vi "SP Convert 2.2 to 3.0 - 3.1.vi"(1 "S Parameter 2.2 Test Parameters":T2={"Tag"="", "Stimulus"={"Use Instrument Settings"=FALSE, "Sweep Type"=enum."Linear", "Sweep"=[{"Fstart, MHz"=500.0, "Fstop, MHz"=1500.0, "Points"=201}], "Blank Frequencies"=FALSE, "Power, dBm"=999.0, "IFBW, Hz"=-1.0, "Sweep Time, s"=-1.0}, "Measurements"=[{"Parameter"=enum."S11", "Channel"=1, "Limits"=[]}], "Reports"={"Reports to Generate"=[], "Print Reports"=FALSE}, "Quick Mode"=FALSE, "Display"={"Retain Settings"=FALSE, "Lock Control"=FALSE, "Plot Orientation"=enum."Single", "CH Controls"=[{"Trace Orientation"=enum."Overlay", "Frequency"={"Start"=500.0, "Stop"=1500.0, "Units"="MHz"}, "CH1Control"={"ChOn"=TRUE, "Measure"=0, "Format"=0, "Autoscale"=TRUE, "Reference"=0.0, "\nRefUnit"="dB/Div", "Position"=5.0, "Scale"=10.0, "ScaleUnit"="dB/Div", "LimitOn"=TRUE, "LimitFill"=FALSE, "Display Data"=0}, "CH2Control"={"ChOn"=TRUE, "Measure"=0, "Format"=0, "Autoscale"=TRUE, "Reference"=0.0, "\nRefUnit"="dB/Div", "Position"=5.0, "Scale"=10.0, "ScaleUnit"="dB/Div", "LimitOn"=TRUE, "LimitFill"=FALSE, "Display Data"=0}}, {"Trace Orientation"=enum."Overlay", "Frequency"={"Start"=500.0, "Stop"=1500.0, "Units"="MHz"}, "CH1Control"={"ChOn"=TRUE, "Measure"=0, "Format"=0, "Autoscale"=TRUE, "Reference"=0.0, "\nRefUnit"="dB/Div", "Position"=5.0, "Scale"=10.0, "ScaleUnit"="dB/Div", "LimitOn"=TRUE, "LimitFill"=FALSE, "Display Data"=0}, "CH2Control"={"ChOn"=TRUE, "Measure"=0, "Format"=0, "Autoscale"=TRUE, "Reference"=0.0, "\nRefUnit"="dB/Div", "Position"=5.0, "Scale"=10.0, "ScaleUnit"="dB/Div", "LimitOn"=TRUE, "LimitFill"=FALSE, "Display Data"=0}}, {"Trace Orientation"=enum."Overlay", "Frequency"={"Start"=500.0, "Stop"=1500.0, "Units"="MHz"}, "CH1Control"={"ChOn"=TRUE, "Measure"=0, "Format"=0, "Autoscale"=TRUE, "Reference"=0.0, "\nRefUnit"="dB/Div", "Position"=5.0, "Scale"=10.0, "ScaleUnit"="dB/Div", "LimitOn"=TRUE, "LimitFill"=FALSE, "Display Data"=0}, "CH2Control"={"ChOn"=TRUE, "Measure"=0, "Format"=0, "Autoscale"=TRUE, "Reference"=0.0, "\nRefUnit"="dB/Div", "Position"=5.0, "Scale"=10.0, "ScaleUnit"="dB/Div", "LimitOn"=TRUE, "LimitFill"=FALSE, "Display Data"=0}}, {"Trace Orientation"=enum."Overlay", "Frequency"={"Start"=500.0, "Stop"=1500.0, "Units"="MHz"}, "CH1Control"={"ChOn"=TRUE, "Measure"=0, "Format"=0, "Autoscale"=TRUE, "Reference"=0.0, "\nRefUnit"="dB/Div", "Position"=5.0, "Scale"=10.0, "ScaleUnit"="dB/Div", "LimitOn"=TRUE, "LimitFill"=FALSE, "Display Data"=0}, "CH2Control"={"ChOn"=TRUE, "Measure"=0, "Format"=0, "Autoscale"=TRUE, "Reference"=0.0, "\nRefUnit"="dB/Div", "Position"=5.0, "Scale"=10.0, "ScaleUnit"="dB/Div", "LimitOn"=TRUE, "LimitFill"=FALSE, "Display Data"=0}}], "Formatted Data"=FALSE}, "Calibrations"=[enum."Not Calibrated", enum."Not Calibrated", enum."Not Calibrated", enum."Not Calibrated"]} {"Display"."CH Controls"."Frequency"."Stop" format="%.3g"; "Display"."CH Controls"."Frequency"."Start" format="%.3g"; "Display"."CH Controls"."CH2Control"."Measure" items=["S11", "S21", "S12", "S22"]; "Display"."CH Controls"."CH2Control"."Reference" format="%#.2g"; "Display"."CH Controls"."CH2Control"."Display Data" items=["Data", "Memory", "Data/Memory"]; "Display"."CH Controls"."CH2Control"."Format" items=["Log Mag", "Phase", "Delay", "Smith", "Polar", "Lin Mag", "SWR", "Loss", "Real", "Imaginary"]; "Display"."CH Controls"."CH2Control"."Scale" min=0.001 step=1.0 format="%#.2g"; "Display"."CH Controls"."CH2Control"."Position" min=0.0 max=10.0; "Display"."CH Controls"."CH1Control"."Measure" items=["S11", "S21", "S12", "S22"]; "Display"."CH Controls"."CH1Control"."Reference" format="%#.2g"; "Display"."CH Controls"."CH1Control"."Display Data" items=["Data", "Memory", "Data/Memory"]; "Display"."CH Controls"."CH1Control"."Format" items=["Log Mag", "Phase", "Delay", "Smith", "Polar", "Lin Mag", "SWR", "Loss", "Real", "Imaginary"]; "Display"."CH Controls"."CH1Control"."Scale" min=0.001 step=1.0 format="%#.2g"; "Display"."CH Controls"."CH1Control"."Position" min=0.0 max=10.0; "Stimulus"."Sweep Time, s" format="%.3g"; "Measurements"."Channel" min=1 max=99 step=1}) -> (0 "S Parameter 3.0 - 3.1 Test Parameters":T1={"Tag"="", "Stimulus"={"Use Instrument Settings"=FALSE, "Sweep Type"=enum."Linear", "Sweep"=[{"Fstart, MHz"=500.0, "Fstop, MHz"=1500.0, "Points"=201}], "Blank Frequencies"=FALSE, "Power, dBm"=999.0, "IFBW, Hz"=-1.0, "Sweep Time, s"=-1.0}, "Measurements"=[], "Reports"={"Reports to Generate"=[], "Print Reports"=FALSE}, "Quick Mode"=FALSE, "Display"={"Retain Settings"=TRUE, "Lock Control"=FALSE, "Plot Orientation"=enum."Single", "CH Controls"=[{"Trace Orientation"=enum."Overlay", "Frequency"={"Start"=500.0, "Stop"=1500.0, "Units"="MHz"}, "CH1Control"={"ChOn"=TRUE, "Measure"=0, "Format"=6, "Autoscale"=FALSE, "Reference"=0.0, "\nRefUnit"="dB/Div", "Position"=5.0, "Scale"=1.0, "ScaleUnit"="dB/Div", "LimitOn"=TRUE, "LimitFill"=FALSE, "Display Data"=0, "Show Markers"=FALSE}, "CH2Control"={"ChOn"=TRUE, "Measure"=0, "Format"=6, "Autoscale"=FALSE, "Reference"=0.0, "\nRefUnit"="dB/Div", "Position"=5.0, "Scale"=1.0, "ScaleUnit"="dB/Div", "LimitOn"=TRUE, "LimitFill"=FALSE, "Display Data"=0, "Show Markers"=FALSE}, "Markers"=[]}, {"Trace Orientation"=enum."Overlay", "Frequency"={"Start"=500.0, "Stop"=1500.0, "Units"="MHz"}, "CH1Control"={"ChOn"=TRUE, "Measure"=0, "Format"=6, "Autoscale"=TRUE, "Reference"=0.0, "\nRefUnit"="dB/Div", "Position"=5.0, "Scale"=1.0, "ScaleUnit"="dB/Div", "LimitOn"=TRUE, "LimitFill"=FALSE, "Display Data"=0, "Show Markers"=FALSE}, "CH2Control"={"ChOn"=TRUE, "Measure"=1, "Format"=0, "Autoscale"=TRUE, "Reference"=0.0, "\nRefUnit"="dB/Div", "Position"=5.0, "Scale"=1.0, "ScaleUnit"="dB/Div", "LimitOn"=TRUE, "LimitFill"=FALSE, "Display Data"=0, "Show Markers"=FALSE}, "Markers"=[]}, {"Trace Orientation"=enum."Overlay", "Frequency"={"Start"=500.0, "Stop"=1500.0, "Units"="MHz"}, "CH1Control"={"ChOn"=TRUE, "Measure"=0, "Format"=6, "Autoscale"=TRUE, "Reference"=0.0, "\nRefUnit"="dB/Div", "Position"=5.0, "Scale"=1.0, "ScaleUnit"="dB/Div", "LimitOn"=TRUE, "LimitFill"=FALSE, "Display Data"=0, "Show Markers"=FALSE}, "CH2Control"={"ChOn"=TRUE, "Measure"=1, "Format"=0, "Autoscale"=TRUE, "Reference"=0.0, "\nRefUnit"="dB/Div", "Position"=5.0, "Scale"=1.0, "ScaleUnit"="dB/Div", "LimitOn"=TRUE, "LimitFill"=FALSE, "Display Data"=0, "Show Markers"=FALSE}, "Markers"=[]}, {"Trace Orientation"=enum."Overlay", "Frequency"={"Start"=500.0, "Stop"=1500.0, "Units"="MHz"}, "CH1Control"={"ChOn"=TRUE, "Measure"=0, "Format"=6, "Autoscale"=TRUE, "Reference"=0.0, "\nRefUnit"="dB/Div", "Position"=5.0, "Scale"=1.0, "ScaleUnit"="dB/Div", "LimitOn"=TRUE, "LimitFill"=FALSE, "Display Data"=0, "Show Markers"=FALSE}, "CH2Control"={"ChOn"=TRUE, "Measure"=1, "Format"=0, "Autoscale"=TRUE, "Reference"=0.0, "\nRefUnit"="dB/Div", "Position"=5.0, "Scale"=1.0, "ScaleUnit"="dB/Div", "LimitOn"=TRUE, "LimitFill"=FALSE, "Display Data"=0, "Show Markers"=FALSE}, "Markers"=[]}], "Formatted Data"=FALSE}, "Calibrations"=[enum."Not Calibrated", enum."Not Calibrated", enum."Not Calibrated", enum."Not Calibrated"]} {"Stimulus"."Sweep Time, s" format="%.3g"; "Display"."CH Controls"."Frequency"."Stop" format="%.3g"; "Display"."CH Controls"."Frequency"."Start" format="%.3g"; "Display"."CH Controls"."CH2Control"."Measure" items=["S11", "S21", "S12", "S22"]; "Display"."CH Controls"."CH2Control"."Reference" format="%#.2g"; "Display"."CH Controls"."CH2Control"."Display Data" items=["Data", "Memory", "Data/Memory"]; "Display"."CH Controls"."CH2Control"."Format" items=["Log Mag", "Phase", "Delay", "Smith", "Polar", "Lin Mag", "SWR", "Loss", "Real", "Imaginary"]; "Display"."CH Controls"."CH2Control"."Scale" min=0.001 step=1.0 format="%#.2g"; "Display"."CH Controls"."CH2Control"."Position" min=0.0 max=10.0; "Display"."CH Controls"."CH1Control"."Measure" items=["S11", "S21", "S12", "S22"]; "Display"."CH Controls"."CH1Control"."Reference" format="%#.2g"; "Display"."CH Controls"."CH1Control"."Display Data" items=["Data", "Memory", "Data/Memory"]; "Display"."CH Controls"."CH1Control"."Format" items=["Log Mag", "Phase", "Delay", "Smith", "Polar", "Lin Mag", "SWR", "Loss", "Real", "Imaginary"]; "Display"."CH Controls"."CH1Control"."Scale" min=0.001 step=1.0 format="%#.2g"; "Display"."CH Controls"."CH1Control"."Position" min=0.0 max=10.0; "Measurements"."Channel" min=1 max=99 step=1; "Measurements"."Limits"."Run" min=1 step=1})   [LabVIEW 2011]
uses:
  TypeDefs/SP Test Parameters v2.2.ctl
  TypeDefs/SP Test Parameters v3.0-3.1.ctl
panel:
  # "Div"
  # "Div"
  # "="
  # "Div"
  # "Div"
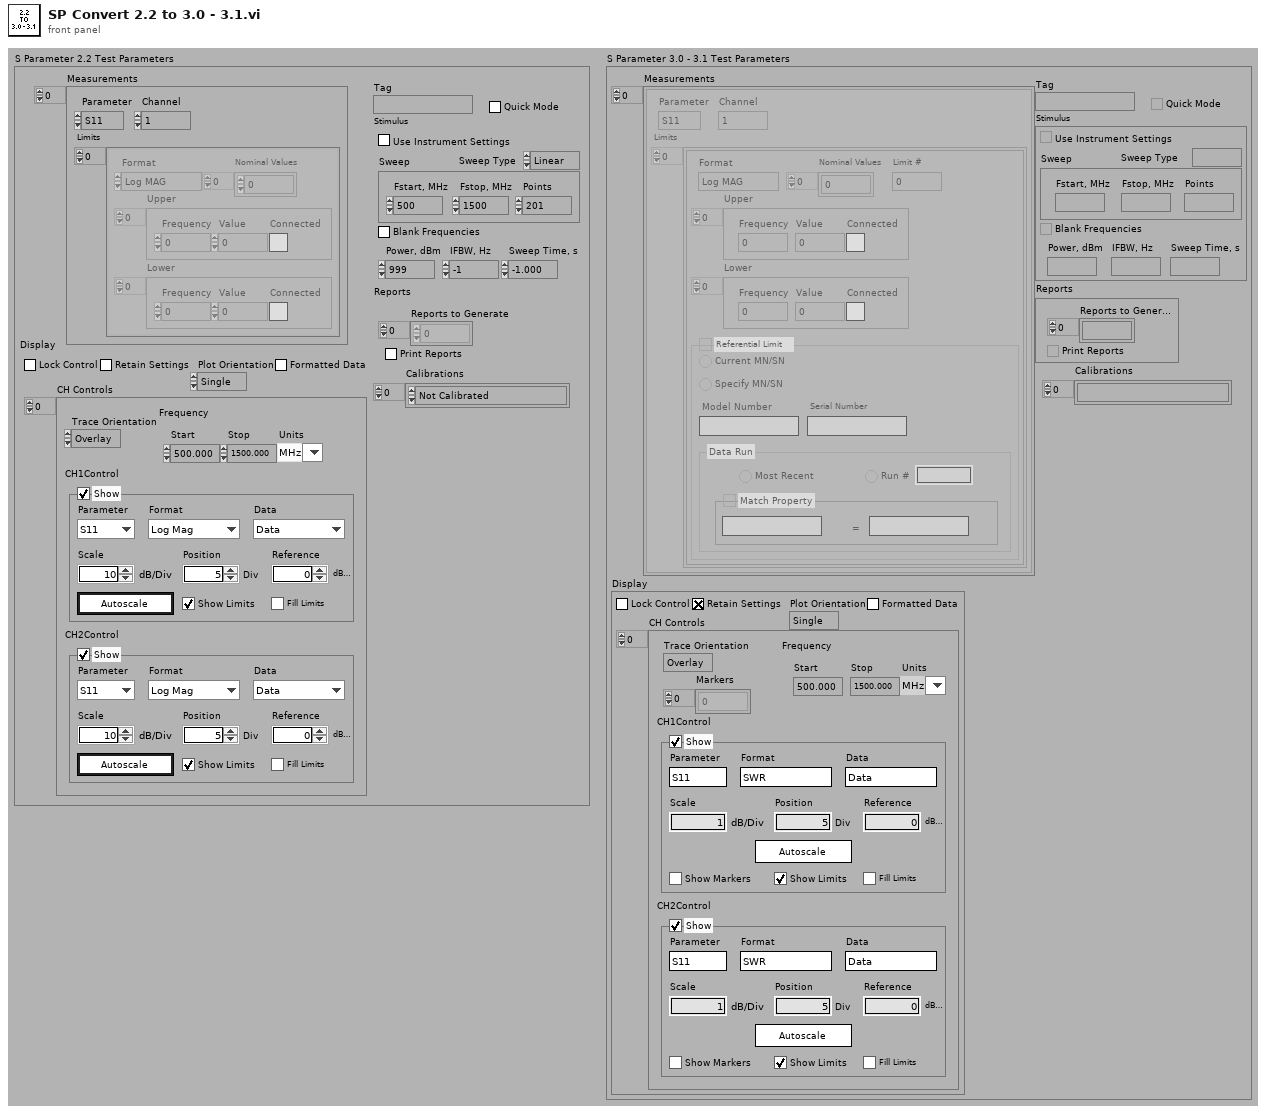
[diagram p1: front panel]
types:
  T1 = typedef "SP Test Parameters v3.0-3.1.ctl" = cluster{"Tag":string, "Stimulus":cluster{"Use Instrument Settings":bool, "Sweep Type":enum32{"Linear", "Log", "List", "Power", "CW"}, "Sweep":cluster{"Fstart, MHz":dbl, "Fstop, MHz":dbl, "Points":i32}[], "Blank Frequencies":bool, "Power, dBm":dbl, "IFBW, Hz":dbl, "Sweep Time, s":dbl}, "Measurements":cluster{"Parameter":enum32{"S11", "S21", "S12", "S22"}, "Channel":i32, "Limits":cluster{"Format":enum16{"Log MAG", "Lin MAG", "VSWR", "Phase", "Delay", "Insertion Loss", "Isolation", "Return Loss"}, "Upper":cluster{"Frequency":dbl, "Value":dbl, "Connected":bool}[], "Lower":cluster{"Frequency":dbl, "Value":dbl, "Connected":bool}[], "Nominal Values":dbl[], "Limit #":i32, "Ref Limit":bool, "Ref Type":enum32{"Current", "Specify"}, "Model":string, "Serial":string, "Run Type":enum32{"Most Recent", "Run #"}, "Run":i32, "Match Property":bool, "Property":string, "Property Value":string}[]}[], "Reports":cluster{"Reports to Generate":i32[], "Print Reports":bool}, "Quick Mode":bool, "Display":cluster{"Retain Settings":bool, "Lock Control":bool, "Plot Orientation":enum32{"Single", "Dual", "Quad"}, "CH Controls":cluster{"Trace Orientation":enum32{"Overlay", "Split"}, "Frequency":cluster{"Start":dbl, "Stop":dbl, "Units":string}, "CH1Control":cluster{"ChOn":bool, "Measure":i32, "Format":i32, "Autoscale":bool, "Reference":dbl, "\nRefUnit":string, "Position":dbl, "Scale":dbl, "ScaleUnit":string, "LimitOn":bool, "LimitFill":bool, "Display Data":u16, "Show Markers":bool}, "CH2Control":cluster{"ChOn":bool, "Measure":i32, "Format":i32, "Autoscale":bool, "Reference":dbl, "\nRefUnit":string, "Position":dbl, "Scale":dbl, "ScaleUnit":string, "LimitOn":bool, "LimitFill":bool, "Display Data":u16, "Show Markers":bool}, "Markers":dbl[]}[], "Formatted Data":bool}, "Calibrations":enum32{"Not Calibrated", "Response", "Response and Isolation", "Full 1-Port (Port 1)", "Full 1-Port (Port 2)", "Full 2-Port", "One Path 2-Port", "TRL/LRM  2-Port", "TOSM Multi-Port", "TOM 2-Port", "TRM 2-Port", "TNA 2-Port"}[]}
  T2 = typedef "SP Test Parameters v2.2.ctl" = cluster{"Tag":string, "Stimulus":cluster{"Use Instrument Settings":bool, "Sweep Type":enum32{"Linear", "Log", "List", "Power", "CW"}, "Sweep":cluster{"Fstart, MHz":dbl, "Fstop, MHz":dbl, "Points":i32}[], "Blank Frequencies":bool, "Power, dBm":dbl, "IFBW, Hz":dbl, "Sweep Time, s":dbl}, "Measurements":cluster{"Parameter":enum32{"S11", "S21", "S12", "S22"}, "Channel":i32, "Limits":cluster{"Format":enum16{"Log MAG", "Lin MAG", "VSWR", "Phase", "Delay", "Insertion Loss", "Isolation", "Return Loss"}, "Upper":cluster{"Frequency":dbl, "Value":dbl, "Connected":bool}[], "Lower":cluster{"Frequency":dbl, "Value":dbl, "Connected":bool}[], "Nominal Values":dbl[]}[]}[], "Reports":cluster{"Reports to Generate":i32[], "Print Reports":bool}, "Quick Mode":bool, "Display":cluster{"Retain Settings":bool, "Lock Control":bool, "Plot Orientation":enum32{"Single", "Dual", "Quad"}, "CH Controls":cluster{"Trace Orientation":enum32{"Overlay", "Split"}, "Frequency":cluster{"Start":dbl, "Stop":dbl, "Units":string}, "CH1Control":cluster{"ChOn":bool, "Measure":i32, "Format":i32, "Autoscale":bool, "Reference":dbl, "\nRefUnit":string, "Position":dbl, "Scale":dbl, "ScaleUnit":string, "LimitOn":bool, "LimitFill":bool, "Display Data":u16}, "CH2Control":cluster{"ChOn":bool, "Measure":i32, "Format":i32, "Autoscale":bool, "Reference":dbl, "\nRefUnit":string, "Position":dbl, "Scale":dbl, "ScaleUnit":string, "LimitOn":bool, "LimitFill":bool, "Display Data":u16}}[], "Formatted Data":bool}, "Calibrations":enum32{"Not Calibrated", "Response", "Response and Isolation", "Full 1-Port (Port 1)", "Full 1-Port (Port 2)", "Full 2-Port", "One Path 2-Port", "TRL/LRM  2-Port", "TOSM Multi-Port", "TOM 2-Port", "TRM 2-Port", "TNA 2-Port"}[]}
  T3 = cluster{"Parameter":enum32{"S11", "S21", "S12", "S22"}, "Channel":i32, "Limits":cluster{"Format":enum16{"Log MAG", "Lin MAG", "VSWR", "Phase", "Delay", "Insertion Loss", "Isolation", "Return Loss"}, "Upper":cluster{"Frequency":dbl, "Value":dbl, "Connected":bool}[], "Lower":cluster{"Frequency":dbl, "Value":dbl, "Connected":bool}[], "Nominal Values":dbl[], "Limit #":i32, "Ref Limit":bool, "Ref Type":enum32{"Current", "Specify"}, "Model":string, "Serial":string, "Run Type":enum32{"Most Recent", "Run #"}, "Run":i32, "Match Property":bool, "Property":string, "Property Value":string}[]}[]
  T4 = cluster{"Trace Orientation":enum32{"Overlay", "Split"}, "Frequency":cluster{"Start":dbl, "Stop":dbl, "Units":string}, "CH1Control":cluster{"ChOn":bool, "Measure":i32, "Format":i32, "Autoscale":bool, "Reference":dbl, "\nRefUnit":string, "Position":dbl, "Scale":dbl, "ScaleUnit":string, "LimitOn":bool, "LimitFill":bool, "Display Data":u16, "Show Markers":bool}, "CH2Control":cluster{"ChOn":bool, "Measure":i32, "Format":i32, "Autoscale":bool, "Reference":dbl, "\nRefUnit":string, "Position":dbl, "Scale":dbl, "ScaleUnit":string, "LimitOn":bool, "LimitFill":bool, "Display Data":u16, "Show Markers":bool}, "Markers":dbl[]}[]
  T5 = cluster{"Parameter":enum32{"S11", "S21", "S12", "S22"}, "Channel":i32, "Limits":cluster{"Format":enum16{"Log MAG", "Lin MAG", "VSWR", "Phase", "Delay", "Insertion Loss", "Isolation", "Return Loss"}, "Upper":cluster{"Frequency":dbl, "Value":dbl, "Connected":bool}[], "Lower":cluster{"Frequency":dbl, "Value":dbl, "Connected":bool}[], "Nominal Values":dbl[], "Limit #":i32, "Ref Limit":bool, "Ref Type":enum32{"Current", "Specify"}, "Model":string, "Serial":string, "Run Type":enum32{"Most Recent", "Run #"}, "Run":i32, "Match Property":bool, "Property":string, "Property Value":string}[]}
  T6 = cluster{"Format":enum16{"Log MAG", "Lin MAG", "VSWR", "Phase", "Delay", "Insertion Loss", "Isolation", "Return Loss"}, "Upper":cluster{"Frequency":dbl, "Value":dbl, "Connected":bool}[], "Lower":cluster{"Frequency":dbl, "Value":dbl, "Connected":bool}[], "Nominal Values":dbl[], "Limit #":i32, "Ref Limit":bool, "Ref Type":enum32{"Current", "Specify"}, "Model":string, "Serial":string, "Run Type":enum32{"Most Recent", "Run #"}, "Run":i32, "Match Property":bool, "Property":string, "Property Value":string}[]
  T7 = cluster{"Parameter":enum32{"S11", "S21", "S12", "S22"}, "Channel":i32, "Limits":cluster{"Format":enum16{"Log MAG", "Lin MAG", "VSWR", "Phase", "Delay", "Insertion Loss", "Isolation", "Return Loss"}, "Upper":cluster{"Frequency":dbl, "Value":dbl, "Connected":bool}[], "Lower":cluster{"Frequency":dbl, "Value":dbl, "Connected":bool}[], "Nominal Values":dbl[]}[]}[]
  T8 = cluster{"Use Instrument Settings":bool, "Sweep Type":enum32{"Linear", "Log", "List", "Power", "CW"}, "Sweep":cluster{"Fstart, MHz":dbl, "Fstop, MHz":dbl, "Points":i32}[], "Blank Frequencies":bool, "Power, dBm":dbl, "IFBW, Hz":dbl, "Sweep Time, s":dbl}
  T9 = cluster{"Reports to Generate":i32[], "Print Reports":bool}
  T10 = enum32{"Not Calibrated", "Response", "Response and Isolation", "Full 1-Port (Port 1)", "Full 1-Port (Port 2)", "Full 2-Port", "One Path 2-Port", "TRL/LRM  2-Port", "TOSM Multi-Port", "TOM 2-Port", "TRM 2-Port", "TNA 2-Port"}[]
  T11 = cluster{"Trace Orientation":enum32{"Overlay", "Split"}, "Frequency":cluster{"Start":dbl, "Stop":dbl, "Units":string}, "CH1Control":cluster{"ChOn":bool, "Measure":i32, "Format":i32, "Autoscale":bool, "Reference":dbl, "\nRefUnit":string, "Position":dbl, "Scale":dbl, "ScaleUnit":string, "LimitOn":bool, "LimitFill":bool, "Display Data":u16}, "CH2Control":cluster{"ChOn":bool, "Measure":i32, "Format":i32, "Autoscale":bool, "Reference":dbl, "\nRefUnit":string, "Position":dbl, "Scale":dbl, "ScaleUnit":string, "LimitOn":bool, "LimitFill":bool, "Display Data":u16}}[]
  T12 = cluster{"Format":enum16{"Log MAG", "Lin MAG", "VSWR", "Phase", "Delay", "Insertion Loss", "Isolation", "Return Loss"}, "Upper":cluster{"Frequency":dbl, "Value":dbl, "Connected":bool}[], "Lower":cluster{"Frequency":dbl, "Value":dbl, "Connected":bool}[], "Nominal Values":dbl[], "Limit #":i32, "Ref Limit":bool, "Ref Type":enum32{"Current", "Specify"}, "Model":string, "Serial":string, "Run Type":enum32{"Most Recent", "Run #"}, "Run":i32, "Match Property":bool, "Property":string, "Property Value":string}
  T13 = cluster{"Format":enum16{"Log MAG", "Lin MAG", "VSWR", "Phase", "Delay", "Insertion Loss", "Isolation", "Return Loss"}, "Upper":cluster{"Frequency":dbl, "Value":dbl, "Connected":bool}[], "Lower":cluster{"Frequency":dbl, "Value":dbl, "Connected":bool}[], "Nominal Values":dbl[]}[]
  T14 = enum16{"Log MAG", "Lin MAG", "VSWR", "Phase", "Delay", "Insertion Loss", "Isolation", "Return Loss"}
  T15 = cluster{"Frequency":dbl, "Value":dbl, "Connected":bool}[]
  T16 = cluster{"Trace Orientation":enum32{"Overlay", "Split"}, "Frequency":cluster{"Start":dbl, "Stop":dbl, "Units":string}, "CH1Control":cluster{"ChOn":bool, "Measure":i32, "Format":i32, "Autoscale":bool, "Reference":dbl, "\nRefUnit":string, "Position":dbl, "Scale":dbl, "ScaleUnit":string, "LimitOn":bool, "LimitFill":bool, "Display Data":u16, "Show Markers":bool}, "CH2Control":cluster{"ChOn":bool, "Measure":i32, "Format":i32, "Autoscale":bool, "Reference":dbl, "\nRefUnit":string, "Position":dbl, "Scale":dbl, "ScaleUnit":string, "LimitOn":bool, "LimitFill":bool, "Display Data":u16, "Show Markers":bool}, "Markers":dbl[]}
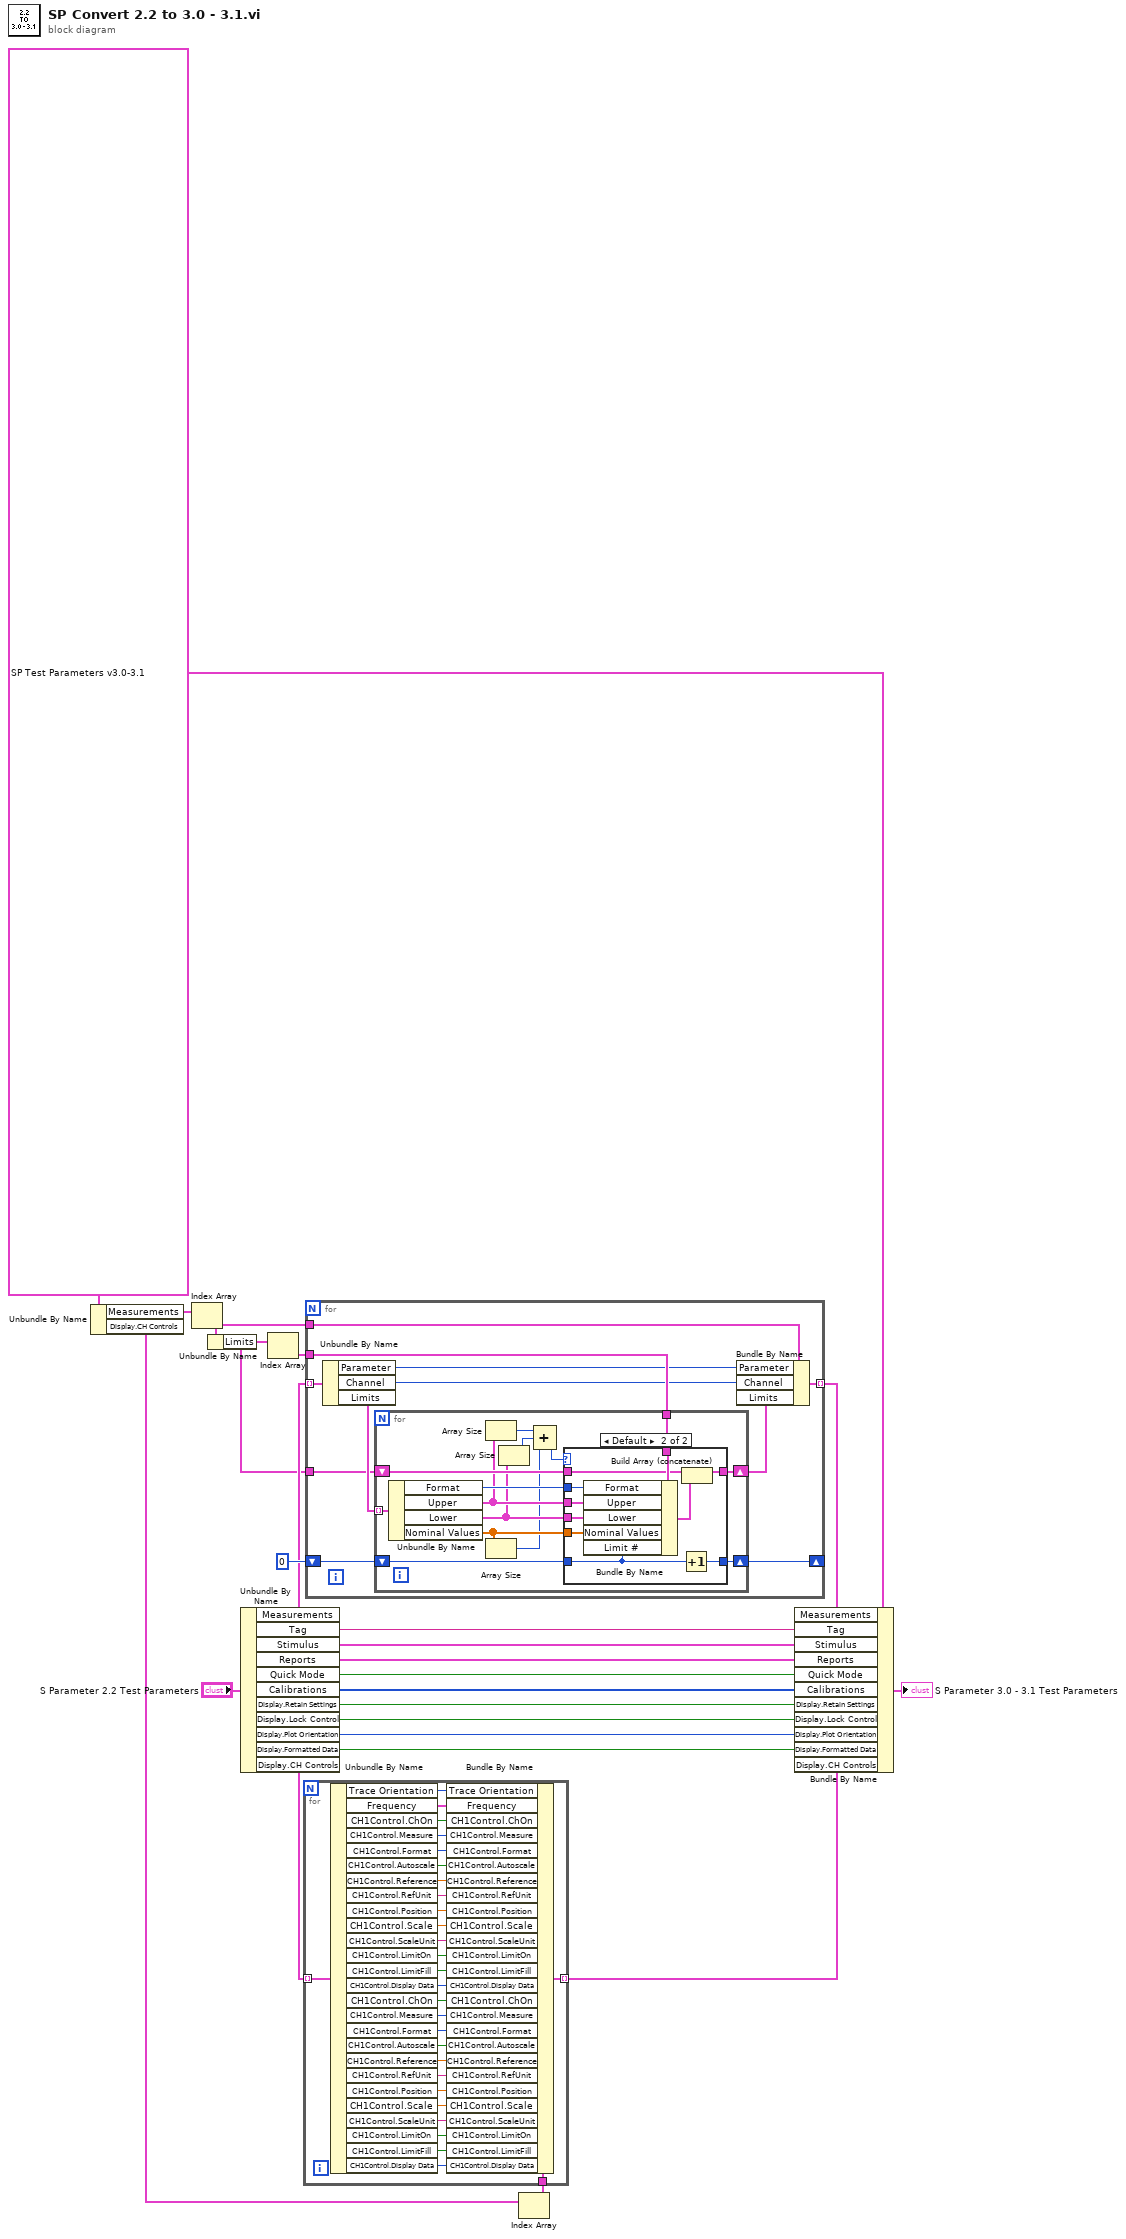
[diagram p0: block diagram]
diagram:
  w4 = T1 {"Tag"="", "Stimulus"={"Use Instrument Settings"=FALSE, "Sweep Type"=enum."Linear", "Sweep"=[{"Fstart, MHz"=500.0, "Fstop, MHz"=1500.0, "Points"=201}], "Blank Frequencies"=FALSE, "Power, dBm"=999.0, "IFBW, Hz"=-1.0, "Sweep Time, s"=-1.0}, "Measurements"=[{"Parameter"=enum."S11", "Channel"=1, "Limits"=[]}, {"Parameter"=enum."S21", "Channel"=2, "Limits"=[]}], "Reports"={"Reports to Generate"=[], "Print Reports"=FALSE}, "Quick Mode"=FALSE, "Display"={"Retain Settings"=TRUE, "Lock Control"=FALSE, "Plot Orientation"=enum."Single", "CH Controls"=[{"Trace Orientation"=enum."Overlay", "Frequency"={"Start"=500.0, "Stop"=1500.0, "Units"="MHz"}, "CH1Control"={"ChOn"=TRUE, "Measure"=0, "Format"=0, "Autoscale"=TRUE, "Reference"=0.0, "\nRefUnit"="dB/Div", "Position"=5.0, "Scale"=10.0, "ScaleUnit"="dB/Div", "LimitOn"=TRUE, "LimitFill"=FALSE, "Display Data"=0, "Show Markers"=FALSE}, "CH2Control"={"ChOn"=TRUE, "Measure"=0, "Format"=0, "Autoscale"=TRUE, "Reference"=0.0, "\nRefUnit"="dB/Div", "Position"=5.0, "Scale"=10.0, "ScaleUnit"="dB/Div", "LimitOn"=TRUE, "LimitFill"=FALSE, "Display Data"=0, "Show Markers"=FALSE}, "Markers"=[]}, {"Trace Orientation"=enum."Overlay", "Frequency"={"Start"=500.0, "Stop"=1500.0, "Units"="MHz"}, "CH1Control"={"ChOn"=TRUE, "Measure"=0, "Format"=0, "Autoscale"=TRUE, "Reference"=0.0, "\nRefUnit"="dB/Div", "Position"=5.0, "Scale"=10.0, "ScaleUnit"="dB/Div", "LimitOn"=TRUE, "LimitFill"=FALSE, "Display Data"=0, "Show Markers"=FALSE}, "CH2Control"={"ChOn"=TRUE, "Measure"=0, "Format"=0, "Autoscale"=TRUE, "Reference"=0.0, "\nRefUnit"="dB/Div", "Position"=5.0, "Scale"=10.0, "ScaleUnit"="dB/Div", "LimitOn"=TRUE, "LimitFill"=FALSE, "Display Data"=0, "Show Markers"=FALSE}, "Markers"=[]}, {"Trace Orientation"=enum."Overlay", "Frequency"={"Start"=500.0, "Stop"=1500.0, "Units"="MHz"}, "CH1Control"={"ChOn"=TRUE, "Measure"=0, "Format"=0, "Autoscale"=TRUE, "Reference"=0.0, "\nRefUnit"="dB/Div", "Position"=5.0, "Scale"=10.0, "ScaleUnit"="dB/Div", "LimitOn"=TRUE, "LimitFill"=FALSE, "Display Data"=0, "Show Markers"=FALSE}, "CH2Control"={"ChOn"=TRUE, "Measure"=0, "Format"=0, "Autoscale"=TRUE, "Reference"=0.0, "\nRefUnit"="dB/Div", "Position"=5.0, "Scale"=10.0, "ScaleUnit"="dB/Div", "LimitOn"=TRUE, "LimitFill"=FALSE, "Display Data"=0, "Show Markers"=FALSE}, "Markers"=[]}, {"Trace Orientation"=enum."Overlay", "Frequency"={"Start"=500.0, "Stop"=1500.0, "Units"="MHz"}, "CH1Control"={"ChOn"=TRUE, "Measure"=0, "Format"=0, "Autoscale"=TRUE, "Reference"=0.0, "\nRefUnit"="dB/Div", "Position"=5.0, "Scale"=10.0, "ScaleUnit"="dB/Div", "LimitOn"=TRUE, "LimitFill"=FALSE, "Display Data"=0, "Show Markers"=FALSE}, "CH2Control"={"ChOn"=TRUE, "Measure"=0, "Format"=0, "Autoscale"=TRUE, "Reference"=0.0, "\nRefUnit"="dB/Div", "Position"=5.0, "Scale"=10.0, "ScaleUnit"="dB/Div", "LimitOn"=TRUE, "LimitFill"=FALSE, "Display Data"=0, "Show Markers"=FALSE}, "Markers"=[]}], "Formatted Data"=FALSE}, "Calibrations"=[enum."Not Calibrated", enum."Not Calibrated", enum."Not Calibrated", enum."Not Calibrated"]} ("S Parameter Test Parameters")
  n1 = Unbundle By Name(w4) -> ("Measurements"=w12:T3, "Display.CH Controls"=w2:T4)
  n2 = Index Array(array=w12) -> (element=w8:T5)  [unwired: 1 in]
  n3 = Unbundle By Name(w8) -> ("Limits"=w7:T6)
  n4 = Unbundle By Name("S Parameter 2.2 Test Parameters") -> ("Measurements"=w10:T7, "Tag"=w21:string, "Stimulus"=w22:T8, "Reports"=w23:T9, "Quick Mode"=w20:bool, "Calibrations"=w19:T10, "Display.Retain Settings"=w16:bool, "Display.Lock Control"=w17:bool, "Display.Plot Orientation"=w18:enum32{"Single", "Dual", "Quad"}, "Display.Formatted Data"=w1:bool, "Display.CH Controls"=w14:T11)
  n5 = Index Array(array=w7) -> (element=w9:T12)  [unwired: 1 in]
  n6 = for {
    tunnel: w10 -> [w34] mode=indexing
    tunnel: w9 -> [w33]
    tunnel: w8 -> [w32]
    tunnel: [w29] -> w6 mode=indexing
    shift-right: [w24] -> _
    shift-left: 0 -> [w28]
    tunnel: w7 -> [w25]
    n7 = Unbundle By Name(w34) -> ("Parameter"=w31:enum32{"S11", "S21", "S12", "S22"}, "Channel"=w30:i32, "Limits"=w27:T13)
    n8 = for {
      tunnel: w27 -> [w48] mode=indexing
      tunnel: w33 -> [w47]
      shift-right: [w43] -> w26
      shift-left: w25 -> [w42]
      shift-right: [w44] -> w24
      shift-left: w28 -> [w45]
      n9 = Unbundle By Name(w48) -> ("Format"=w46:T14, "Upper"=w40:T15, "Lower"=w39:T15, "Nominal Values"=w41:dbl[])
      n10 = Array Size(array=w40) -> (size(s)=w38:i32)
      n11 = Array Size(array=w41) -> (size(s)=w36:i32)
      n12 = Array Size(array=w39) -> (size(s)=w37:i32)
      n13 = Compound Arithmetic op=ADD(w38, w37, w36) -> (w35:i32)
      n14 = case shown="Default" w35 {
        tunnel: w47 -> [_ w60]
        tunnel: w46 -> [_ w59]
        tunnel: w40 -> [_ w58]
        tunnel: w39 -> [_ w57]
        tunnel: w41 -> [_ w56]
        tunnel: w45 -> [w49 w51]
        tunnel: [w49 w52] -> w44
        tunnel: [w50 w54] -> w43
        tunnel: w42 -> [w50 w53]
        frame 0 {
        }
        frame Default {
          n15 = Bundle By Name(cluster=w60, "Format"=w59, "Upper"=w58, "Lower"=w57, "Nominal Values"=w56, "Limit #"=w51) -> (w55:T12)
          n16 = Increment(x=w51) -> (x+1=w52:i32)
          n17 = Build Array (concatenate)(w53, w55) -> (w54:T6)
        }
      }
    }
    n18 = Bundle By Name(cluster=w32, "Parameter"=w31, "Channel"=w30, "Limits"=w26) -> (w29:T5)
  }
  n19 = Index Array(array=w2) -> (element=w15:T16)  [unwired: 1 in]
  n20 = for {
    tunnel: w14 -> [w89] mode=indexing
    tunnel: w15 -> [w88]
    tunnel: [w85] -> w13 mode=indexing
    n21 = Unbundle By Name(w89) -> ("Trace Orientation"=w86:enum32{"Overlay", "Split"}, "Frequency"=w87:cluster{"Start":dbl, "Stop":dbl, "Units":string}, "CH1Control.ChOn"=w84:bool, "CH1Control.Measure"=w83:i32, "CH1Control.Format"=w82:i32, "CH1Control.Autoscale"=w81:bool, "CH1Control.Reference"=w80:dbl, "CH1Control.RefUnit"=w79:string, "CH1Control.Position"=w78:dbl, "CH1Control.Scale"=w77:dbl, "CH1Control.ScaleUnit"=w76:string, "CH1Control.LimitOn"=w75:bool, "CH1Control.LimitFill"=w74:bool, "CH1Control.Display Data"=w73:u16, "CH1Control.ChOn"=w72:bool, "CH1Control.Measure"=w71:i32, "CH1Control.Format"=w69:i32, "CH1Control.Autoscale"=w70:bool, "CH1Control.Reference"=w68:dbl, "CH1Control.RefUnit"=w67:string, "CH1Control.Position"=w66:dbl, "CH1Control.Scale"=w65:dbl, "CH1Control.ScaleUnit"=w64:string, "CH1Control.LimitOn"=w63:bool, "CH1Control.LimitFill"=w62:bool, "CH1Control.Display Data"=w61:u16)
    n22 = Bundle By Name(cluster=w88, "Trace Orientation"=w86, "Frequency"=w87, "CH1Control.ChOn"=w84, "CH1Control.Measure"=w83, "CH1Control.Format"=w82, "CH1Control.Autoscale"=w81, "CH1Control.Reference"=w80, "CH1Control.RefUnit"=w79, "CH1Control.Position"=w78, "CH1Control.Scale"=w77, "CH1Control.ScaleUnit"=w76, "CH1Control.LimitOn"=w75, "CH1Control.LimitFill"=w74, "CH1Control.Display Data"=w73, "CH1Control.ChOn"=w72, "CH1Control.Measure"=w71, "CH1Control.Format"=w69, "CH1Control.Autoscale"=w70, "CH1Control.Reference"=w68, "CH1Control.RefUnit"=w67, "CH1Control.Position"=w66, "CH1Control.Scale"=w65, "CH1Control.ScaleUnit"=w64, "CH1Control.LimitOn"=w63, "CH1Control.LimitFill"=w62, "CH1Control.Display Data"=w61) -> (w85:T16)
  }
  n23 = Bundle By Name(cluster=w4, "Measurements"=w6, "Tag"=w21, "Stimulus"=w22, "Reports"=w23, "Quick Mode"=w20, "Calibrations"=w19, "Display.Retain Settings"=w16, "Display.Lock Control"=w17, "Display.Plot Orientation"=w18, "Display.Formatted Data"=w1, "Display.CH Controls"=w13) -> (→"S Parameter 3.0 - 3.1 Test Parameters":T1)
